vi "Error Handler.vi"(8 "error in (no error)":errorcluster, 10 "state":T1=enum."Start", 11 "Dispatcher in":refnum<class "Dispatcher Thread.lvclass">) -> (0 "error out":errorcluster, 3 "Dispatcher out":refnum<class "Dispatcher Thread.lvclass">)   [LabVIEW 2017, in "DSF Core.lvlib" / "Dispatcher Thread.lvclass"]
uses:
  Dispatcher Thread.lvclass
  C:/Git/DSF/Core/Classes/Thread/Thread.lvclass
  Interface/Dispatcher/Command.ctl
  Thread.lvclass/Thread.ctl
  <vilib>/NI/Memory Manager/Classes/Pointer/Pointer.lvclass/Pointer.ctl
  Dispatcher Thread.lvclass/Dispatcher Thread.ctl
  Get Error Pointer.vi
  <vilib>/NI/Memory Manager/Classes/Pointer/Get Address.vi
  Write Error Pointer.vi
  Pointers/Error/Error Pointer.lvclass
  C:/Program Files (x86)/National Instruments/LabVIEW 2017/vi.lib/NI/Memory Manager/Classes/Pointer/Pointer.lvclass
  Pointers/Error/Write Error Pointer.vi
  Interface/Logging/Send.vi
  Interface/Logging/Send Logging Command.vi
  Interface/Dispatcher/Dispatcher Interface.lvclass
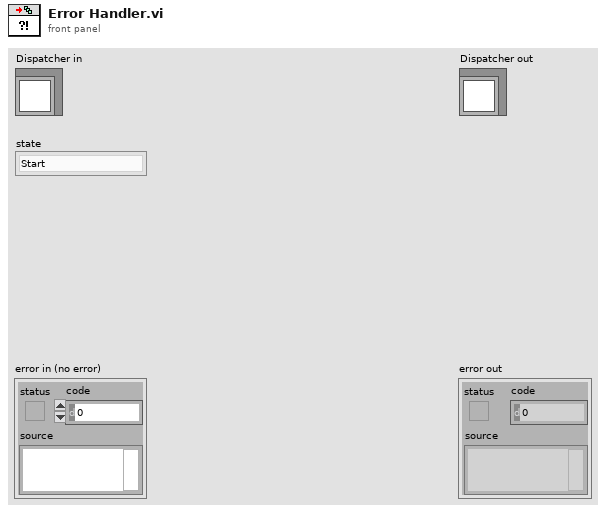
[diagram p1: front panel]
types:
  T1 = typedef "DSF Core.lvlib/Dispatcher Interface.lvclass/Command.ctl" = enum8{"Idle", "Start", "Rx", "Tx", "Set Inline Buffer", "Shutdown"}
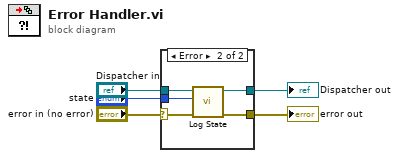
[diagram p0: block diagram]
diagram:
  n1 = case shown="Error" "error in (no error)" {
    selector: "error in (no error)" -> [w7 w11]
    tunnel: [w7 w10] -> w5
    tunnel: "Dispatcher in" -> [w6 w12]
    tunnel: [w6 w9] -> w4
    tunnel: "state" -> [_ w8]
    frame No Error {
    }
    frame Error {
      n2 = call "Log State.vi"("error in (no error)"=w11, "state"=w8, "Dispatcher in"=w12) -> ("error out"=w10:errorcluster, "Dispatcher out"=w9:refnum<class "Dispatcher Thread.lvclass">)  [unwired: 7 in]
    }
  }
  "error out" <- w5
  "Dispatcher out" <- w4
